vi "main_v3.0.vi"() -> ()   [LabVIEW 2017]
uses:
  <vilib>/addons/database/Connection.llb/DB Tools Open Connec (String).vi
  <vilib>/addons/database/Auxilliary.llb/DB Tools Format Datetime String (Time Stamp).vi
  <vilib>/addons/database/_DB Variant To Data/Database Variant To Data.xnode
  <vilib>/addons/database/NI_Database_API.lvlib
  kernel32.dll
panel:
  out "Table":string[][](table)
  out "query for userID":string="WHERE  user_ID =  100000000"
  in  "user_ID_eachSensor":string(combo)
  in  "delete_user_fromsensor_btn":bool
  in  "add_user_tosensor_btn":bool
  in  "sensor_ID_forSensors":string(combo)
  in  "user_ID_forUsers":string(combo)
  in  "delete_user_btn":bool
  in  "delete_sensor_btn":bool
  in  "user_ID_forSensors":string(combo)
  in  "sensor_ID_forAlerts":string(combo)
  in  "alert_receiver":string
  in  "alert_code":string
  in  "add_alert_btn":bool
  in  "sensor_description":string
  in  "sensor_enabled_state":string(combo)="True"
  in  "sensor_longitude":string
  in  "sensor_latitude":string
  in  "sensor_label":string
  in  "user_permission":string(combo)="User"
  in  "user_groupID":string(combo)="Group1"
  in  "user_phone":string
  in  "user_email":string
  in  "user_lastname":string
  in  "user_firstname":string
  in  "add_sensor_btn":bool
  out "error out":errorcluster
  in  "error in (no error)":errorcluster
  out "Unix time":dbl=1703036813.2194657 format="%#_13g"
  in  "add_user_btn":bool
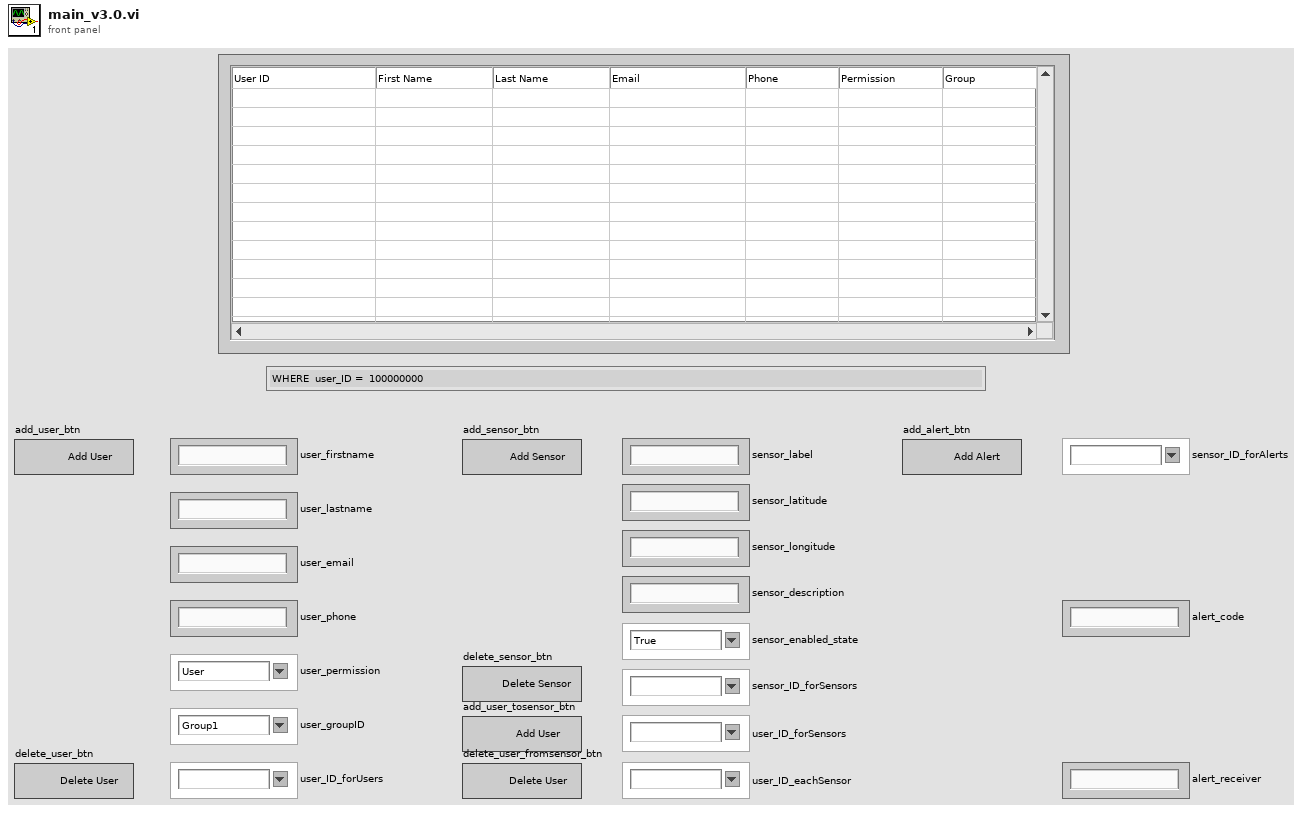
[diagram p1: front panel]
types:
  T1 = typedef "NI_Database_API.lvlib/Conn ObjectReference.ctl" = refnum<k1>
  T2 = cluster{string, "user_firstname":string, "user_lastname":string, "user_email":string, "user_phone":string, "user_permission":string, "user_groupID":string}
  T3 = cluster{string, "sensor_label":string, "sensor_latitude":string, "sensor_longitude":string, "sensor_description":string, "sensor_enabled_state":string, "table":string}
  T4 = cluster{"Unix time":dbl, "sensor_ID_forAlerts":string, "date/time string":string, "alert_code":string, "alert_receiver":string}
  T5 = cluster{"[0]":u16, "[1]":u16, "[2]":u16, "[3]":u16, "[4]":u16, "[5]":u16, "[6]":u16, "[7]":u16, "[8]":u16, "[9]":u16, "[10]":u16, "[11]":u16, "[12]":u16, "[13]":u16, "[14]":u16, "[15]":u16, "[16]":u16, "[17]":u16, "[18]":u16, "[19]":u16, "[20]":u16, "[21]":u16, "[22]":u16, "[23]":u16, "[24]":u16, "[25]":u16, "[26]":u16, "[27]":u16, "[28]":u16, "[29]":u16, "[30]":u16, "[31]":u16, "[32]":u16, "[33]":u16, "[34]":u16, "[35]":u16, "[36]":u16, "[37]":u16, "[38]":u16, "[39]":u16, "[40]":u16, "[41]":u16, "[42]":u16, "[43]":u16, "[44]":u16, "[45]":u16, "[46]":u16, "[47]":u16, "[48]":u16, "[49]":u16, "[50]":u16, "[51]":u16, "[52]":u16, "[53]":u16, "[54]":u16, "[55]":u16, "[56]":u16, "[57]":u16, "[58]":u16, "[59]":u16, "[60]":u16, "[61]":u16, "[62]":u16, "[63]":u16, "[64]":u16, "[65]":u16, "[66]":u16, "[67]":u16, "[68]":u16, "[69]":u16, "[70]":u16, "[71]":u16, "[72]":u16, "[73]":u16, "[74]":u16, "[75]":u16, "[76]":u16, "[77]":u16, "[78]":u16, "[79]":u16, "[80]":u16, "[81]":u16, "[82]":u16, "[83]":u16, "[84]":u16, "[85]":u16}
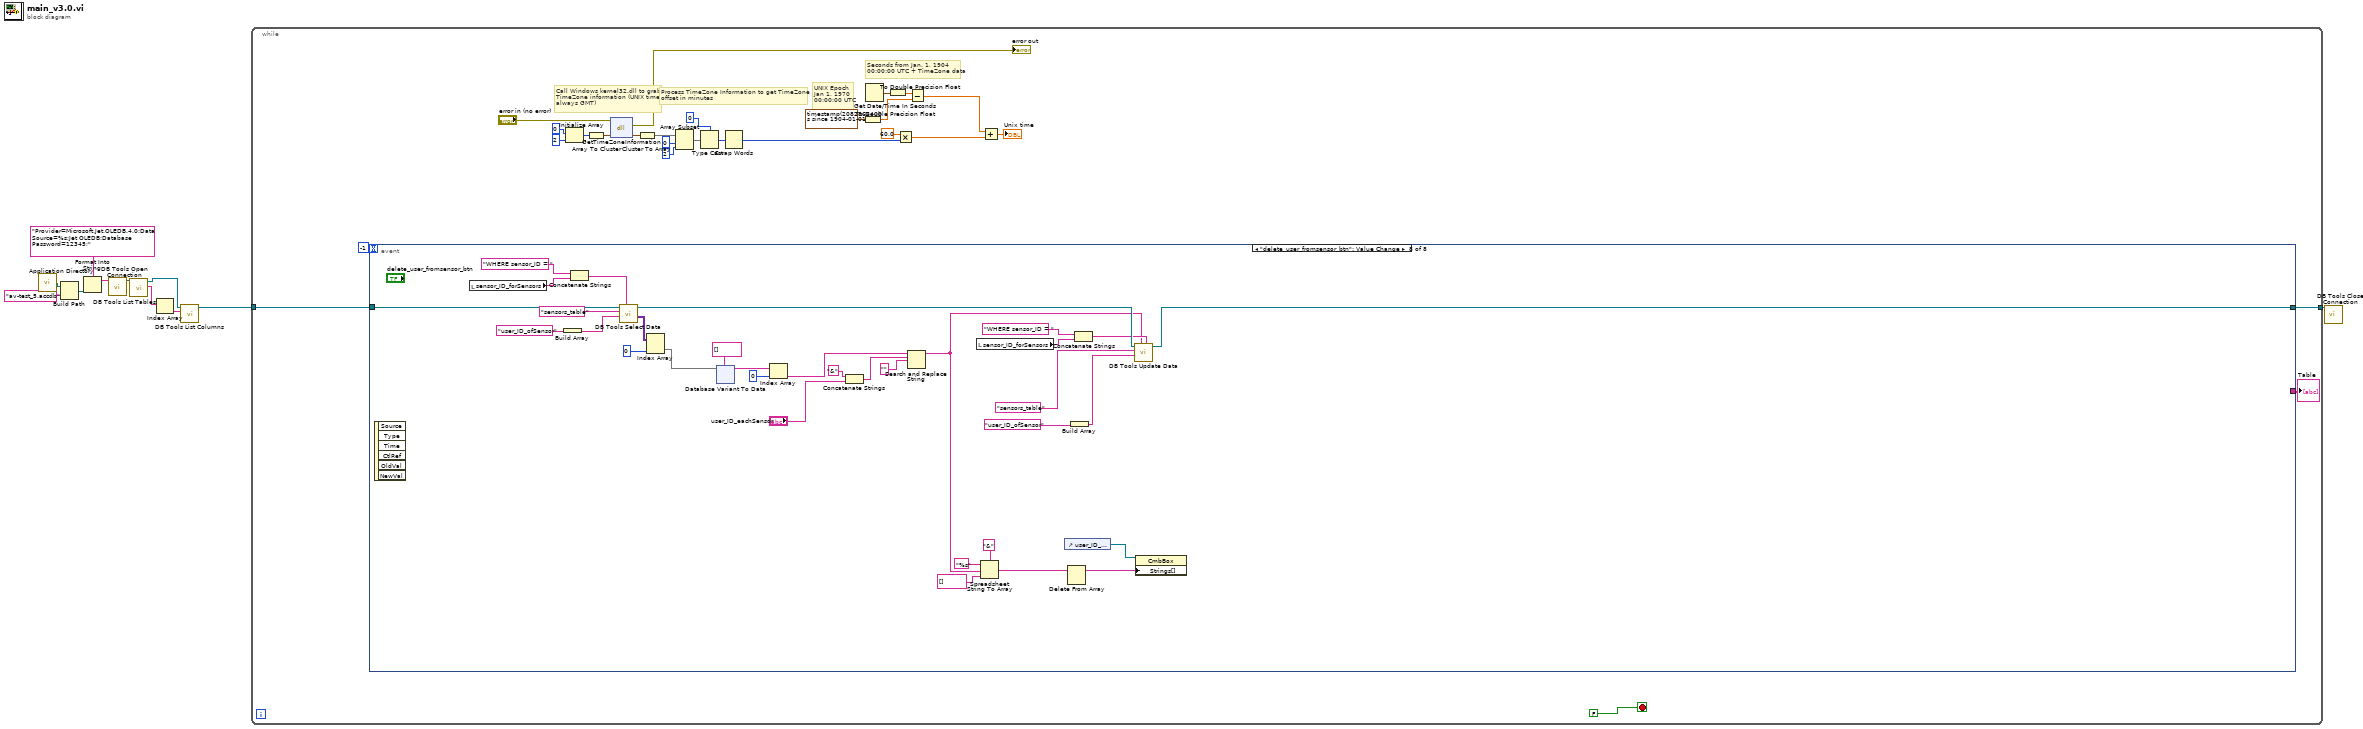
[diagram p0: block diagram]
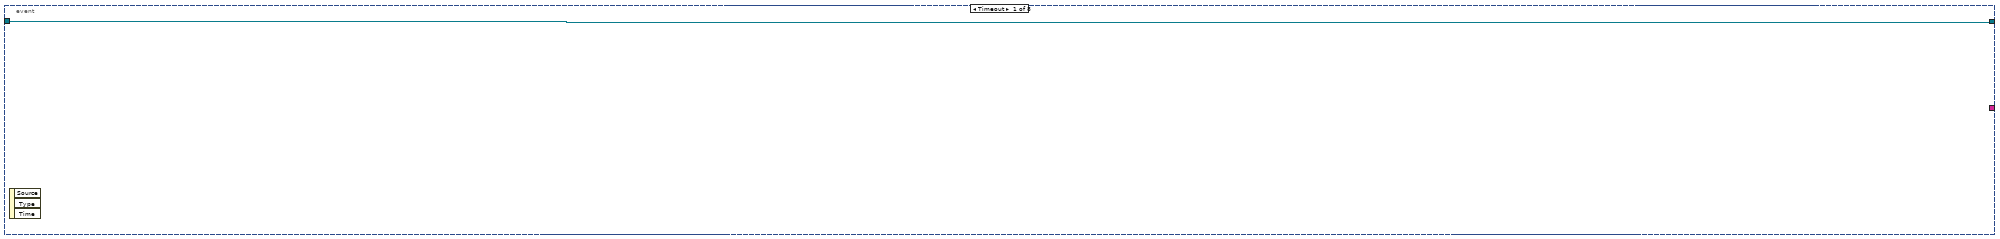
[diagram p2: hidden frame]
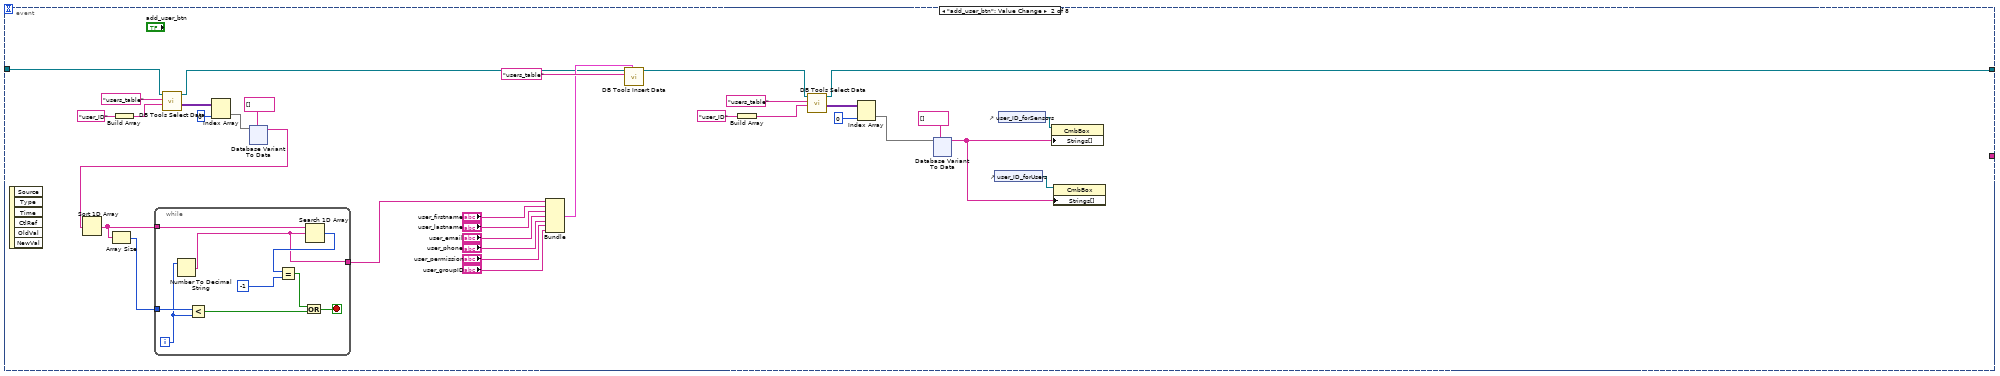
[diagram p3: hidden frame]
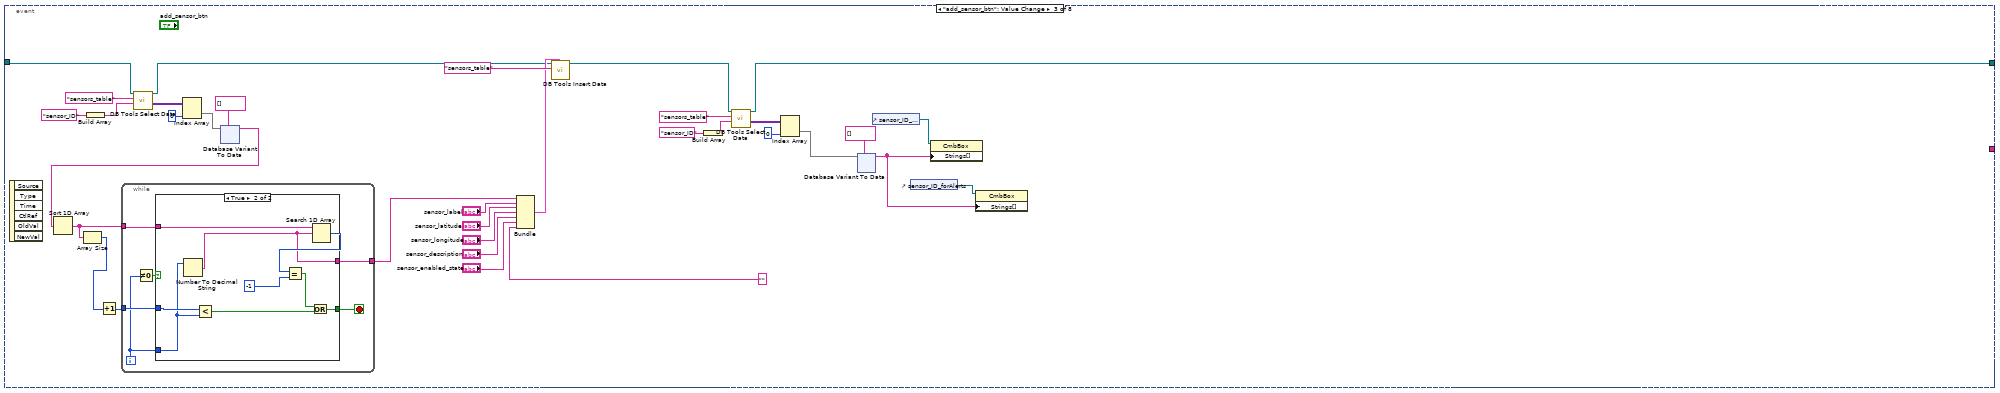
[diagram p4: hidden frame]
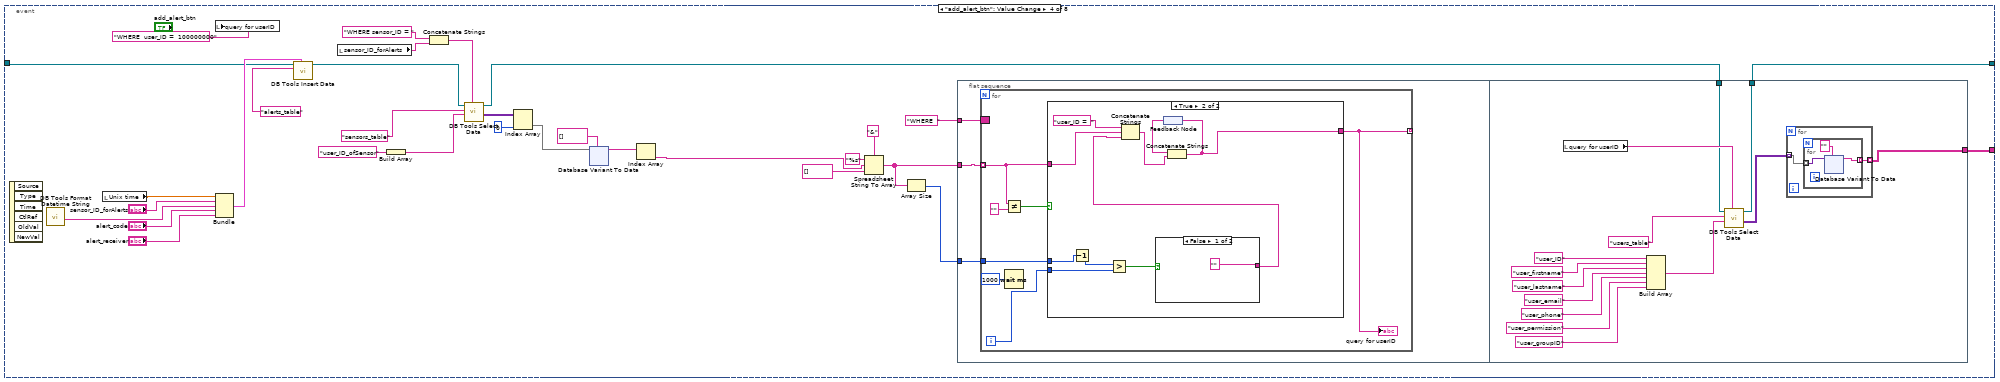
[diagram p6: hidden frame]
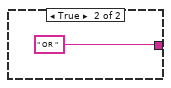
[diagram p8: hidden frame]
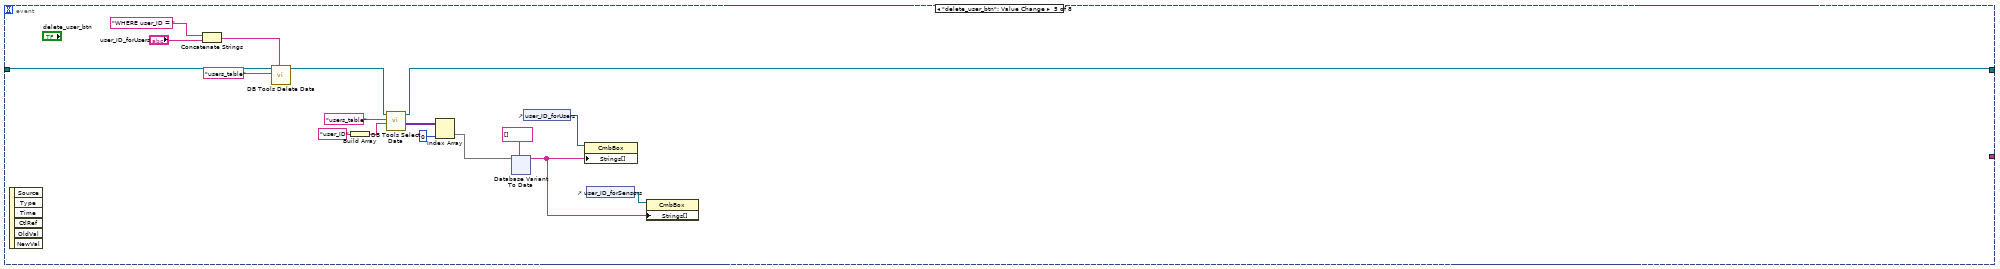
[diagram p9: hidden frame]
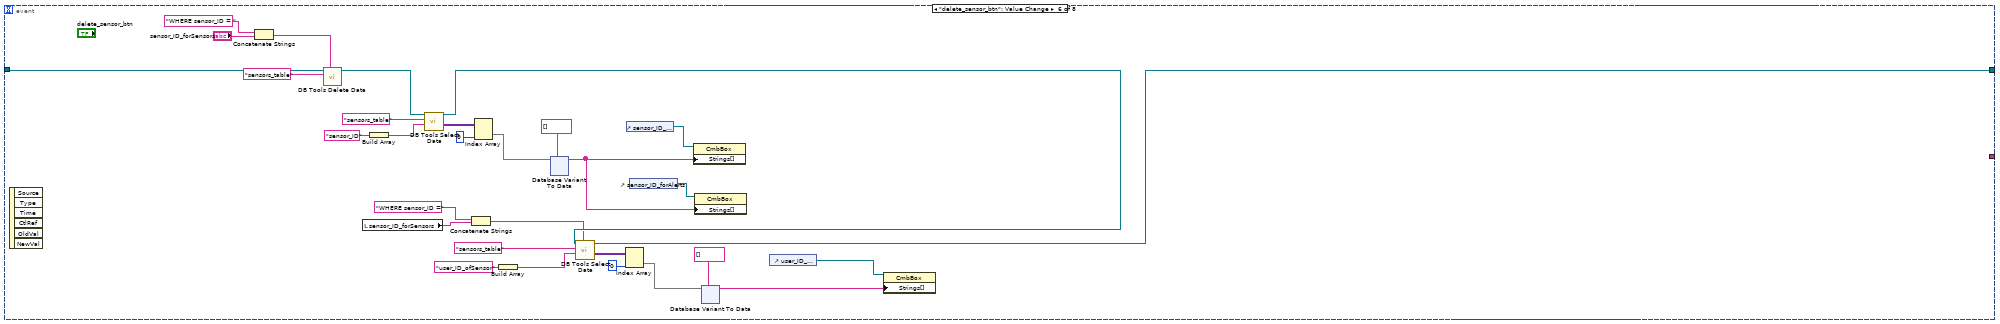
[diagram p10: hidden frame]
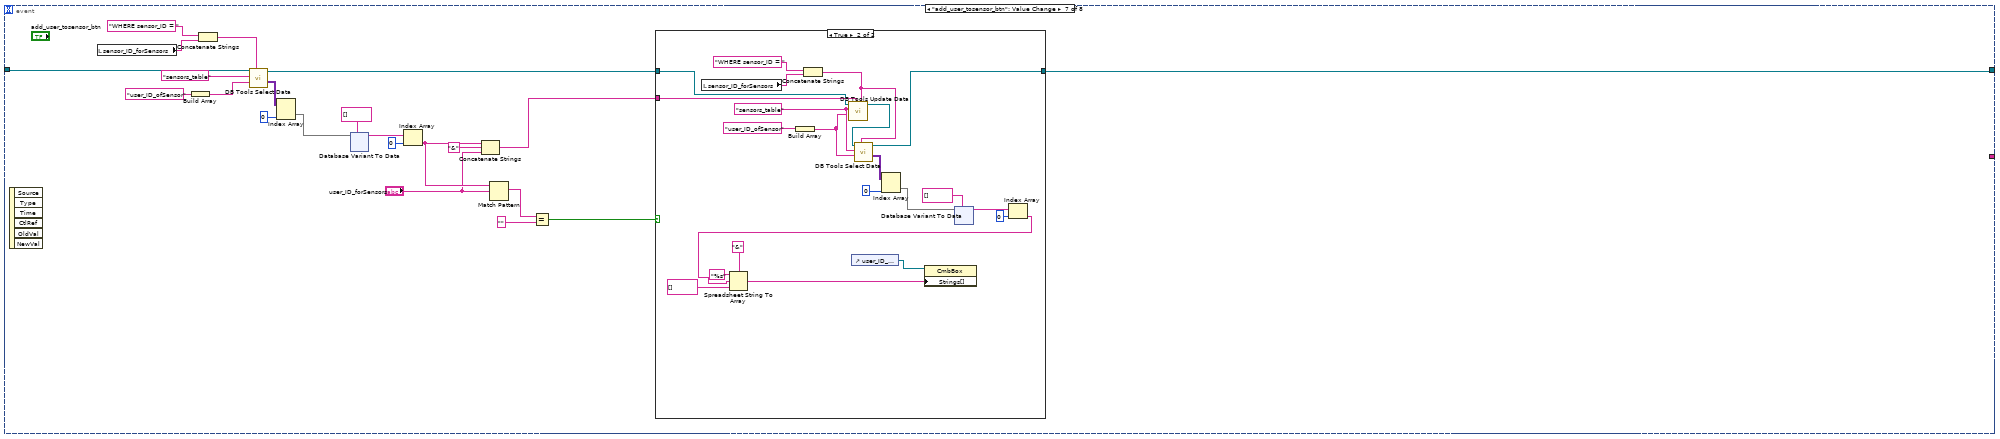
[diagram p11: hidden frame]
diagram:
  n1 = call <vilib>:"Application Directory.vi"() -> ("Application Directory"=w10:path)
  n2 = Build Path(base path=w10, name or relative path="av-test_5.accdb" ("table")) -> (appended path=w8:path)
  n3 = Format Into String(format string="Provider=Microsoft.Jet.OLEDB.4.0;Data Source=%s;Jet OLEDB:Database Password=12345;", w8) -> (resulting string=w7:string)  [unwired: 2 in, 1 out]
  n4 = call-poly <vilib>:"DB Tools Open Connection.vi"("connection information"=w7) -> ("connection reference"=w3:T1)  [unwired: 7 in, 1 out]
  n5 = call <vilib>:"DB Tools List Tables.vi"("connection reference"=w3) -> ("tables"=w6:string[], "connection reference out"=w4:T1)  [unwired: 4 in, 1 out]
  n6 = Index Array(array=w6) -> (element=w5:string)  [unwired: 1 in]
  n7 = call <vilib>:"DB Tools List Columns.vi"("table"=w5, "connection reference"=w4) -> ("connection reference out"=w2:T1)  [unwired: 2 in, 3 out]
  n8 = while {
    tunnel: w2 -> [w38]
    tunnel: [w37] -> w1
    stop <- FALSE stop-if-true
    # "Seconds from Jan. 1, 1904\n00:00:00 UTC + TimeZone data"
    # "UNIX Epoch\nJan 1, 1970\n00:00:00 UTC"
    # "Process TimeZone Information to get TimeZone\noffset in minutes"
    # "Call Windows kernel32.dll to grab\nTimeZone information (UNIX time\nalways GMT)"
    n9 = event shown="[7] \"delete_user_fromsensor_btn\": Value Change" {
      selector: _ -> [_ _ _ _ _ _ _ _]
      dyn-events: _ -> [_ _ _ _ _ _ _ _]
      timeout: -1 -> [_ _ _ _ _ _ _ _]
      tunnel: w38 -> [w39 w42 w162 w311 w437 w505 w603 w715]
      tunnel: [w39 w53 w173 w292 w426 w484 w586 w710] -> w37
      tunnel: [_ _ _ w290 _ _ _ _] -> w12
      event Timeout {
        n10 = event-data() -> ()  [unwired: 1 in, 3 out]
      }
      event "add_user_btn": Value Change {
        n11 = event-data() -> ()  [unwired: 1 in, 6 out]
        n12 = Build Array("user_ID" ("table")) -> (w50:string[])
        n13 = call <vilib>:"DB Tools Select Data.vi"("columns"=w50, "table"="users_table", "connection reference"=w42) -> ("data"=w49:variant[][], "connection reference out"=w41:T1)  [unwired: 3 in, 1 out]
        n14 = Index Array(array=w49, index (col)=0 ("disabled index (col)")) -> (element=w48:variant[])  [unwired: 1 in]
        n15 = xnode "Database Variant To Data"("database variant"=w48, "type"=string[] []) -> ("data"=w43:string[])  [unwired: 1 in, 1 out]
        n16 = Sort 1D Array(array=w43) -> (sorted array=w52:string[])
        n17 = Array Size(array=w52) -> (size(s)=w51:i32)
        n18 = while {
          tunnel: w52 -> [w119]
          tunnel: w51 -> [w118]
          tunnel: [w111] -> w40
          i -> [w115]
          stop <- w116 stop-if-true
          n19 = Number To Decimal String(number=w115) -> (decimal integer string=w111:string)  [unwired: 1 in]
          n20 = Less?(x=w118, y=w115) -> (x < y?=w117:bool)
          n21 = Search 1D Array(1D array=w119, element=w111) -> (index of element=w114:i32)  [unwired: 1 in]
          n22 = Equal?(x=w114, y=-1) -> (x = y?=w112:bool)
          n23 = Or(x=w112, y=w117) -> (x .or. y?=w116:bool)
        }
        n24 = Bundle(w40, "user_firstname"="user_firstname", "user_lastname"="user_lastname", "user_email"="user_email", "user_phone"="user_phone", "user_permission"="user_permission", "user_groupID"="user_groupID") -> (w71:T2)  [unwired: 1 in]
        n25 = call <vilib>:"DB Tools Insert Data.vi"("data"=w71, "table"="users_table", "connection reference"=w41) -> ("connection reference out"=w56:T1)  [unwired: 7 in, 1 out]
        n26 = Build Array("user_ID" ("table")) -> (w64:string[])
        n27 = call <vilib>:"DB Tools Select Data.vi"("columns"=w64, "table"="users_table", "connection reference"=w56) -> ("data"=w63:variant[][], "connection reference out"=w53:T1)  [unwired: 3 in, 1 out]
        n28 = Index Array(array=w63, index (col)=0 ("disabled index (col)")) -> (element=w62:variant[])  [unwired: 1 in]
        n29 = xnode "Database Variant To Data"("database variant"=w62, "type"=string[] []) -> ("data"=w54:string[])  [unwired: 1 in, 1 out]
        n30 = control-ref of="user_ID_forUsers"() -> (w55:refnum<vi>)
        n31 = control-ref of="user_ID_forSensors"() -> (w61:refnum<vi>)
        n32 = property on="Property Node" class="CmbBox"(reference=w61, "Strings[]"=w54) -> ()  [unwired: 1 in, 2 out]
        n33 = property on="Property Node" class="CmbBox"(reference=w55, "Strings[]"=w54) -> ()  [unwired: 1 in, 2 out]
      }
      event "add_sensor_btn": Value Change {
        n34 = event-data() -> ()  [unwired: 1 in, 6 out]
        n35 = Build Array("sensor_ID" ("table")) -> (w170:string[])
        n36 = call <vilib>:"DB Tools Select Data.vi"("columns"=w170, "table"="sensors_table", "connection reference"=w162) -> ("data"=w169:variant[][], "connection reference out"=w161:T1)  [unwired: 3 in, 1 out]
        n37 = Index Array(array=w169, index (col)=0 ("disabled index (col)")) -> (element=w168:variant[])  [unwired: 1 in]
        n38 = xnode "Database Variant To Data"("database variant"=w168, "type"=string[] []) -> ("data"=w163:string[])  [unwired: 1 in, 1 out]
        n39 = Sort 1D Array(array=w163) -> (sorted array=w171:string[])
        n40 = Array Size(array=w171) -> (size(s)=w158:i32)
        n41 = Increment(x=w158) -> (x+1=w159:i32)
        n42 = while {
          tunnel: w171 -> [w235]
          tunnel: w159 -> [w234]
          tunnel: [w232] -> w160
          i -> [w230]
          stop <- w233 stop-if-true
          n43 = Not Equal To 0?(x=w230) -> (x != 0?=w231:bool)
          n44 = case shown="True" w231 {
            tunnel: w235 -> [_ w244]
            tunnel: w234 -> [_ w243]
            tunnel: [_ w241] -> w233
            tunnel: [_ w237] -> w232
            tunnel: w230 -> [_ w236]
            frame False {
            }
            frame True {
              n45 = Number To Decimal String(number=w236) -> (decimal integer string=w237:string)  [unwired: 1 in]
              n46 = Less?(x=w243, y=w236) -> (x < y?=w242:bool)
              n47 = Search 1D Array(1D array=w244, element=w237) -> (index of element=w240:i32)  [unwired: 1 in]
              n48 = Equal?(x=w240, y=-1) -> (x = y?=w238:bool)
              n49 = Or(x=w238, y=w242) -> (x .or. y?=w241:bool)
            }
          }
        }
        n50 = Bundle(w160, "sensor_label"="sensor_label", "sensor_latitude"="sensor_latitude", "sensor_longitude"="sensor_longitude", "sensor_description"="sensor_description", "sensor_enabled_state"="sensor_enabled_state", "table"="") -> (w190:T3)  [unwired: 1 in]
        n51 = call <vilib>:"DB Tools Insert Data.vi"("data"=w190, "table"="sensors_table", "connection reference"=w161) -> ("connection reference out"=w177:T1)  [unwired: 7 in, 1 out]
        n52 = Build Array("sensor_ID" ("table")) -> (w184:string[])
        n53 = call <vilib>:"DB Tools Select Data.vi"("columns"=w184, "table"="sensors_table", "connection reference"=w177) -> ("data"=w183:variant[][], "connection reference out"=w173:T1)  [unwired: 3 in, 1 out]
        n54 = Index Array(array=w183, index (col)=0 ("disabled index (col)")) -> (element=w182:variant[])  [unwired: 1 in]
        n55 = xnode "Database Variant To Data"("database variant"=w182, "type"=string[] []) -> ("data"=w172:string[])  [unwired: 1 in, 1 out]
        n56 = control-ref of="sensor_ID_forSensors"() -> (w175:refnum<vi>)
        n57 = control-ref of="sensor_ID_forAlerts"() -> (w176:refnum<vi>)
        n58 = property on="Property Node" class="CmbBox"(reference=w175, "Strings[]"=w172) -> ()  [unwired: 1 in, 2 out]
        n59 = property class="CmbBox"(reference=w176, "Strings[]"=w172) -> ()  [unwired: 1 in, 2 out]
      }
      event "add_alert_btn": Value Change {
        n60 = event-data() -> ()  [unwired: 1 in, 6 out]
        n61 = call-poly <vilib>:"DB Tools Format Datetime String.vi"() -> ("date/time string"=w309:string)  [unwired: 1 in]
        n62 = local read "Unix time"() -> (w310:dbl)
        n63 = local write "query for userID"("WHERE  user_ID =  100000000" ("query for userID")) -> ()
        n64 = Bundle("Unix time"=w310, "sensor_ID_forAlerts"="sensor_ID_forAlerts", "date/time string"=w309, "alert_code"="alert_code", "alert_receiver"="alert_receiver") -> (w312:T4)  [unwired: 1 in]
        n65 = call <vilib>:"DB Tools Insert Data.vi"("data"=w312, "table"="alerts_table", "connection reference"=w311) -> ("connection reference out"=w294:T1)  [unwired: 7 in, 1 out]
        n66 = local read "sensor_ID_forAlerts"() -> (w297:string)
        n67 = Build Array("user_ID_ofSensor" ("table")) -> (w305:string[])
        n68 = Concatenate Strings("WHERE sensor_ID = " ("format string"), w297) -> (w296:string)
        n69 = call <vilib>:"DB Tools Select Data.vi"("condition"=w296, "columns"=w305, "table"="sensors_table", "connection reference"=w294) -> ("data"=w304:variant[][], "connection reference out"=w293:T1)  [unwired: 2 in, 1 out]
        n70 = Index Array(array=w304, index (col)=0 ("disabled index (col)")) -> (element=w303:variant[])  [unwired: 1 in]
        n71 = xnode "Database Variant To Data"("database variant"=w303, "type"=string[] []) -> ("data"=w295:string[])  [unwired: 1 in, 1 out]
        n72 = Index Array(array=w295) -> (element=w291:string)  [unwired: 1 in]
        n73 = Spreadsheet String To Array(delimiter (Tab)="&", format string="%s", spreadsheet string=w291, array type (2D Dbl)=string[] []) -> (array=w285:string[])
        n74 = Array Size(array=w285) -> (size(s)=w284:i32)
        n75 = flat-sequence {
          tunnel: "WHERE  " -> [w316]
          tunnel: w285 -> [w315]
          tunnel: w284 -> [w314]
          tunnel: w293 -> [w345]
          tunnel: [w344] -> w292
          tunnel: [w336] -> w290
          frame #0 {
            n76 = for {
              tunnel: w315 -> [w323] mode=indexing
              border: w316 -> [_]
              tunnel: [w320] -> _ mode=indexing
              tunnel: w314 -> [w318]
              i -> [w317]
              n77 = Wait (ms)(milliseconds to wait=u32 1000) -> ()  [unwired: 1 out]
              n78 = Not Equal?(x=w323, y="") -> (x != y?=w321:bool)
              n79 = case shown="True" w321 {
                tunnel: w323 -> [_ w332]
                tunnel: [_ w330] -> w320
                tunnel: w318 -> [_ w327]
                tunnel: w317 -> [_ w328]
                frame False {
                }
                frame True {
                  n80 = Decrement(x=w327) -> (x-1=w326:i32)
                  n81 = Greater?(x=w326, y=w328) -> (0:w325:bool)
                  n82 = case shown="False" w325 {
                    tunnel: ["" ("string") " OR " ("string")] -> w324
                    frame False {
                    }
                    frame True {
                    }
                  }
                  n83 = Concatenate Strings("user_ID =  " ("string"), w332, w324) -> (w329:string)
                  n84 = feedback #1() -> (w333:string)
                  n85 = Concatenate Strings(w333, w329) -> (w330:string)
                  n86 = feedback-in #1(w330) -> ()
                }
              }
              "query for userID" <- w320
            }
          }
          frame #1 {
            n87 = local read "query for userID"() -> (w346:string)
            n88 = Build Array("user_ID" ("table"), "user_firstname" ("table"), "user_lastname" ("table"), "user_email" ("table"), "user_phone" ("table"), "user_permission" ("table"), "user_groupID" ("table")) -> (w349:string[])
            n89 = call <vilib>:"DB Tools Select Data.vi"("condition"=w346, "columns"=w349, "table"="users_table", "connection reference"=w345) -> ("data"=w343:variant[][], "connection reference out"=w344:T1)  [unwired: 2 in, 1 out]
            n90 = for {
              tunnel: w343 -> [w351] mode=indexing
              tunnel: [w350] -> w336 mode=indexing
              n91 = for {
                tunnel: [w353] -> w350 mode=indexing
                tunnel: w351 -> [w352] mode=indexing
                n92 = xnode "Database Variant To Data"("database variant"=w352, "type"="") -> ("data"=w353:string)  [unwired: 1 in, 1 out]
              }
            }
          }
        }
      }
      event "delete_user_btn": Value Change {
        n93 = event-data() -> ()  [unwired: 1 in, 6 out]
        n94 = Concatenate Strings("WHERE user_ID = " ("format string"), "user_ID_forUsers") -> (w438:string)
        n95 = call <vilib>:"DB Tools Delete Data.vi"("condition"=w438, "table"="users_table", "connection reference"=w437) -> ("connection reference out"=w429:T1)  [unwired: 7 in, 1 out]
        n96 = Build Array("user_ID" ("table")) -> (w436:string[])
        n97 = call <vilib>:"DB Tools Select Data.vi"("columns"=w436, "table"="users_table", "connection reference"=w429) -> ("data"=w435:variant[][], "connection reference out"=w426:T1)  [unwired: 3 in, 1 out]
        n98 = Index Array(array=w435, index (col)=0 ("disabled index (col)")) -> (element=w434:variant[])  [unwired: 1 in]
        n99 = xnode "Database Variant To Data"("database variant"=w434, "type"=string[] []) -> ("data"=w425:string[])  [unwired: 1 in, 1 out]
        n100 = control-ref of="user_ID_forUsers"() -> (w428:refnum<vi>)
        n101 = property on="Property Node" class="CmbBox"(reference=w428, "Strings[]"=w425) -> ()  [unwired: 1 in, 2 out]
        n102 = control-ref of="user_ID_forSensors"() -> (w427:refnum<vi>)
        n103 = property on="Property Node" class="CmbBox"(reference=w427, "Strings[]"=w425) -> ()  [unwired: 1 in, 2 out]
      }
      event "delete_sensor_btn": Value Change {
        n104 = event-data() -> ()  [unwired: 1 in, 6 out]
        n105 = Concatenate Strings("WHERE sensor_ID = " ("format string"), "sensor_ID_forSensors") -> (w507:string)
        n106 = call <vilib>:"DB Tools Delete Data.vi"("condition"=w507, "table"="sensors_table", "connection reference"=w505) -> ("connection reference out"=w497:T1)  [unwired: 7 in, 1 out]
        n107 = local read "sensor_ID_forSensors"() -> (w481:string)
        n108 = Build Array("sensor_ID" ("table")) -> (w504:string[])
        n109 = call <vilib>:"DB Tools Select Data.vi"("columns"=w504, "table"="sensors_table", "connection reference"=w497) -> ("data"=w503:variant[][], "connection reference out"=w485:T1)  [unwired: 3 in, 1 out]
        n110 = Concatenate Strings("WHERE sensor_ID =" ("format string"), w481) -> (w483:string)
        n111 = Index Array(array=w503, index (col)=0 ("disabled index (col)")) -> (element=w502:variant[])  [unwired: 1 in]
        n112 = Build Array("user_ID_ofSensor" ("table")) -> (w493:string[])
        n113 = xnode "Database Variant To Data"("database variant"=w502, "type"=string[] []) -> ("data"=w495:string[])  [unwired: 1 in, 1 out]
        n114 = call <vilib>:"DB Tools Select Data.vi"("condition"=w483, "columns"=w493, "table"="sensors_table", "connection reference"=w485) -> ("data"=w492:variant[][], "connection reference out"=w484:T1)  [unwired: 2 in, 1 out]
        n115 = Index Array(array=w492, index (col)=0 ("disabled index (col)")) -> (element=w491:variant[])  [unwired: 1 in]
        n116 = control-ref of="sensor_ID_forSensors"() -> (w496:refnum<vi>)
        n117 = control-ref of="sensor_ID_forAlerts"() -> (w494:refnum<vi>)
        n118 = property on="Property Node" class="CmbBox"(reference=w496, "Strings[]"=w495) -> ()  [unwired: 1 in, 2 out]
        n119 = property on="Property Node" class="CmbBox"(reference=w494, "Strings[]"=w495) -> ()  [unwired: 1 in, 2 out]
        n120 = xnode "Database Variant To Data"("database variant"=w491, "type"=string[] []) -> ("data"=w487:string[])  [unwired: 1 in, 1 out]
        n121 = control-ref of="user_ID_eachSensor"() -> (w486:refnum<vi>)
        n122 = property on="Property Node" class="CmbBox"(reference=w486, "Strings[]"=w487) -> ()  [unwired: 1 in, 2 out]
      }
      event "add_user_tosensor_btn": Value Change {
        n123 = event-data() -> ()  [unwired: 1 in, 6 out]
        n124 = local read "sensor_ID_forSensors"() -> (w607:string)
        n125 = Build Array("user_ID_ofSensor" ("table")) -> (w602:string[])
        n126 = Concatenate Strings("WHERE sensor_ID = " ("format string"), w607) -> (w604:string)
        n127 = call <vilib>:"DB Tools Select Data.vi"("condition"=w604, "columns"=w602, "table"="sensors_table", "connection reference"=w603) -> ("data"=w597:variant[][], "connection reference out"=w587:T1)  [unwired: 2 in, 1 out]
        n128 = Index Array(array=w597, index (col)=0 ("disabled index (col)")) -> (element=w600:variant[])  [unwired: 1 in]
        n129 = xnode "Database Variant To Data"("database variant"=w600, "type"=string[] []) -> ("data"=w596:string[])  [unwired: 1 in, 1 out]
        n130 = Index Array(array=w596, index=0) -> (element=w593:string)
        n131 = Concatenate Strings(w593, "&" ("string"), "user_ID_forSensors") -> (w588:string)
        n132 = Match Pattern(string=w593, regular expression="user_ID_forSensors") -> (match substring=w591:string)  [unwired: 1 in, 3 out]
        n133 = Equal?(x=w591, y="") -> (x = y?=w589:bool)
        n134 = case shown="True" w589 {
          tunnel: w588 -> [_ w626]
          tunnel: w587 -> [_ w625]
          tunnel: [_ w615] -> w586
          frame False {
          }
          frame True {
            w613 = "sensors_table" ("table")
            n135 = local read "sensor_ID_forSensors"() -> (w629:string)
            n136 = Build Array("user_ID_ofSensor" ("table")) -> (w612:string[])
            n137 = Concatenate Strings("WHERE sensor_ID = " ("format string"), w629) -> (w614:string)
            n138 = call <vilib>:"DB Tools Update Data.vi"("condition"=w614, "data"=w626, "columns"=w612, "table"=w613, "connection reference"=w625) -> ("connection reference out"=w616:T1)  [unwired: 5 in, 1 out]
            n139 = control-ref of="user_ID_eachSensor"() -> (w610:refnum<vi>)
            n140 = call <vilib>:"DB Tools Select Data.vi"("condition"=w614, "columns"=w612, "table"=w613, "connection reference"=w616) -> ("data"=w619:variant[][], "connection reference out"=w615:T1)  [unwired: 2 in, 1 out]
            n141 = Index Array(array=w619, index (col)=0 ("disabled index (col)")) -> (element=w622:variant[])  [unwired: 1 in]
            n142 = xnode "Database Variant To Data"("database variant"=w622, "type"=string[] []) -> ("data"=w618:string[])  [unwired: 1 in, 1 out]
            n143 = Index Array(array=w618, index=0) -> (element=w611:string)
            n144 = Spreadsheet String To Array(delimiter (Tab)="&", format string="%s", spreadsheet string=w611, array type (2D Dbl)=string[] []) -> (array=w608:string[])
            n145 = property on="Property Node" class="CmbBox"(reference=w610, "Strings[]"=w608) -> ()  [unwired: 1 in, 2 out]
          }
        }
      }
      event "delete_user_fromsensor_btn": Value Change {
        n146 = event-data() -> ()  [unwired: 1 in, 6 out]
        n147 = local read "sensor_ID_forSensors"() -> (w724:string)
        n148 = Build Array("user_ID_ofSensor" ("table")) -> (w726:string[])
        n149 = Concatenate Strings("WHERE sensor_ID = " ("format string"), w724) -> (w728:string)
        n150 = call <vilib>:"DB Tools Select Data.vi"("condition"=w728, "columns"=w726, "table"="sensors_table", "connection reference"=w715) -> ("data"=w731:variant[][], "connection reference out"=w711:T1)  [unwired: 2 in, 1 out]
        n151 = Index Array(array=w731, index (col)=0 ("disabled index (col)")) -> (element=w734:variant[])  [unwired: 1 in]
        n152 = xnode "Database Variant To Data"("database variant"=w734, "type"=string[] []) -> ("data"=w730:string[])  [unwired: 1 in, 1 out]
        n153 = Index Array(array=w730, index=0) -> (element=w720:string)
        n154 = Concatenate Strings("&" ("string"), "user_ID_eachSensor") -> (w719:string)
        n155 = Search and Replace String(input string=w720, search string=w719, replace string="" ("replace string (\"\")")) -> (result string=w706:string)  [unwired: 5 in, 3 out]
        n156 = local read "sensor_ID_forSensors"() -> (w713:string)
        n157 = Spreadsheet String To Array(delimiter (Tab)="&", format string="%s", spreadsheet string=w706, array type (2D Dbl)=string[] []) -> (array=w723:string[])
        n158 = control-ref of="user_ID_eachSensor"() -> (w716:refnum<vi>)
        n159 = Delete From Array(array=w723) -> (array with subset deleted=w717:string[])  [unwired: 2 in, 1 out]
        n160 = Build Array("user_ID_ofSensor" ("table")) -> (w707:string[])
        n161 = Concatenate Strings("WHERE sensor_ID = " ("format string"), w713) -> (w709:string)
        n162 = call <vilib>:"DB Tools Update Data.vi"("condition"=w709, "data"=w706, "columns"=w707, "table"="sensors_table", "connection reference"=w711) -> ("connection reference out"=w710:T1)  [unwired: 5 in, 1 out]
        n163 = property on="Property Node" class="CmbBox"(reference=w716, "Strings[]"=w717) -> ()  [unwired: 1 in, 2 out]
      }
    }
    "Table" <- w12
    n164 = Initialize Array(u16 0 ("element"), 2 ("dimension size")) -> (w33:u16[])
    n165 = Array To Cluster(array=w33) -> (cluster=w30:T5)
    n166 = dll-call lib="kernel32.dll" fn="GetTimeZoneInformation"(error in="error in (no error)", "lpTimeZoneInformation"=w30) -> (error out=→"error out":errorcluster, "lpTimeZoneInformation"=w29:T5)  [unwired: 2 in, 2 out]
    n167 = Cluster To Array(cluster=w29) -> (array=w28:u16[])
    n168 = Array Subset(array=w28, index=0, length=2) -> (w24:u16[])
    n169 = Type Cast(type=0, x=w24) -> (*(type *) &x=w23:i32)
    n170 = Swap Words(1:w23) -> (0:w19:i32)
    n171 = To Double Precision Float(number=timestamp(2082866400 s since 1904-01-01)) -> (double precision float=w34:dbl)
    n172 = Get Date/Time In Seconds() -> (seconds since 1Jan1904=w13:timestamp)
    n173 = To Double Precision Float(number=w13) -> (double precision float=w15:dbl)
    n174 = Multiply(x=60.0 ("y"), y=w19) -> (x*y=w20:dbl)
    n175 = Subtract(x=w15, y=w34) -> (x-y=w21:dbl)
    n176 = Add(x=w21, y=w20) -> (x+y=→"Unix time":dbl)
  }
  n177 = call <vilib>:"DB Tools Close Connection.vi"("connection reference"=w1) -> ()  [unwired: 6 in, 1 out]
